vi "StrafeCalc.vi"(6 "WheelHoldButton":bool, 7 "CurrentAngle":dbl, 8 "JoystickY":dbl, 9 "JoystickX":dbl) -> (0 "LeftVelocity":dbl, 1 "RightVelocity":dbl, 2 "DesiredAngle 2":dbl, 3 "DesiredAngle1":dbl)   [LabVIEW 2011]
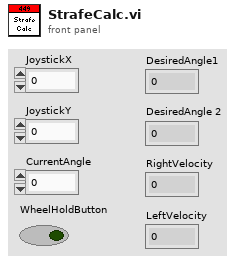
[diagram p1: front panel]
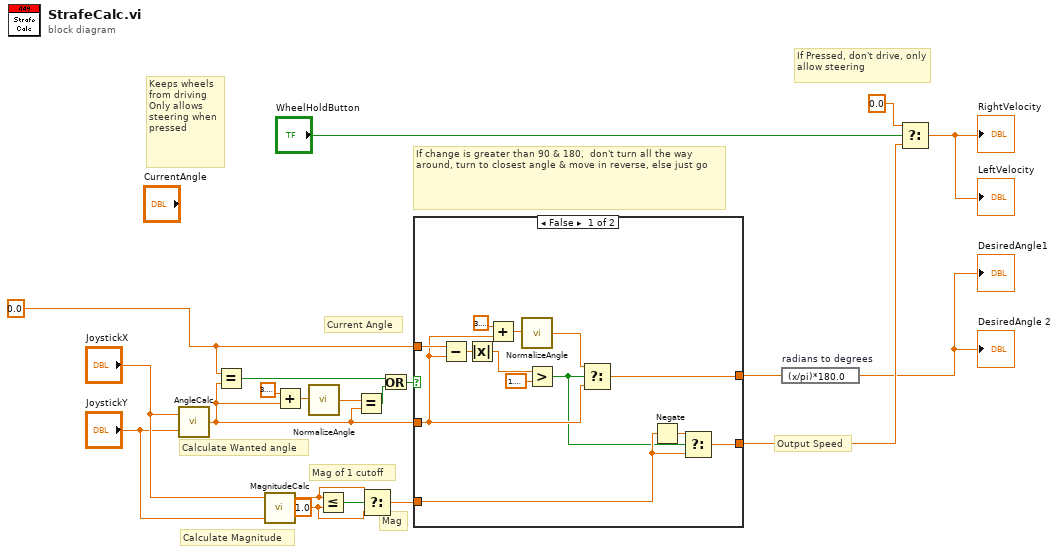
[diagram p0: block diagram]
diagram:
  w11 = 1.0 ("y")
  w20 = 0.0 ("Angle")
  # "If change is greater than 90 & 180,  don't turn all the way around, turn to closest angle & move in reverse, else just go"
  # "Current Angle"
  # "Mag of 1 cutoff"
  # "Mag"
  # "Output Speed"
  # "Calculate Magnitude"
  # "Calculate Wanted angle"
  # "If Pressed, don't drive, only allow steering"
  # "Keeps wheels\nfrom driving\nOnly allows\nsteering when\npressed"
  n1 = call "AngleCalc.vi"("Y"="JoystickY", "X"="JoystickX") -> ("Angle"=w3:dbl)
  n2 = Equal?(x=w20, y=w3) -> (x = y?=w4:bool)
  n3 = call "MagnitudeCalc.vi"("Y"="JoystickY", "X"="JoystickX") -> ("sqrt(X^2+Y^2)"=w10:dbl)  [unwired: 3 in]
  n4 = Add(x=3.141592653589793, y=w3) -> (x+y=w2:dbl)
  n5 = call "NormalizeAngle.vi"("Angle"=w2) -> ("AngleFrom(0-360)"=w1:dbl)
  n6 = Less Or Equal?(x=w10, y=w11) -> (x <= y?=w12:bool)
  n7 = Equal?(x=w1, y=w3) -> (x = y?=w5:bool)
  n8 = Select(t=w10, s=w12, f=w11) -> (s? t:f=w13:dbl)
  n9 = Or(x=w4, y=w5) -> (x .or. y?=w6:bool)
  n10 = case shown="False" w6 {
    tunnel: w20 -> [w27 w34]
    tunnel: [w29 w34] -> w8
    tunnel: w13 -> [w30 w35]
    tunnel: w3 -> [w24 _]
    tunnel: [w33 w35] -> w14
    frame False {
      n11 = Subtract(x=w27, y=w24) -> (x-y=w32:dbl)
      n12 = Absolute Value(x=w32) -> (abs(x)=w22:dbl)
      n13 = Add(x=3.141592653589793, y=w24) -> (x+y=w25:dbl)
      n14 = call "NormalizeAngle.vi"("Angle"=w25) -> ("AngleFrom(0-360)"=w23:dbl)
      n15 = Greater?(x=w22, y=1.5707963267948966) -> (0:w21:bool)
      n16 = Select(t=w23, s=w21, f=w24) -> (s? t:f=w29:dbl)
      n17 = Negate(x=w30) -> (-x=w31:dbl)
      n18 = Select(t=w31, s=w21, f=w30) -> (s? t:f=w33:dbl)
    }
    frame True {
      # "If they are equal, don't care"
    }
  }
  n19 = expression code="(x/pi)*180.0" "radians to degrees"(w8) -> (→"DesiredAngle1" →"DesiredAngle 2":dbl)
  n20 = Select(t=0.0, s="WheelHoldButton", f=w14) -> (s? t:f=→"RightVelocity" →"LeftVelocity":dbl)
